vi "driveMotionProfile.vi"() -> ()   [LabVIEW 2018]
doc: "This VI is called for each TeleOp packet received from the DS where the robot is not disabled. It is often used to read from the joysticks and update I/O or to update setpoints for timed control loops. It should complete and return within 20 milliseconds or it may miss DS packets."
uses:
  Motion Profile SM.ctl
  <vilib>/Rock Robotics/WPI/ThirdParty/Phoenix-LabVIEW/Pigeon IMU/CTRE_PigeonIMU_CalibrationMode.ctl
  <vilib>/Rock Robotics/WPI/ThirdParty/Phoenix-LabVIEW/Motor Controller/Controls/CTRE_Phoenix_MotorControl_ControlMode.ctl
  <vilib>/Rock Robotics/WPI/ThirdParty/Phoenix-LabVIEW/Motor Controller/Controls/CTRE_Phoenix_MotorControl_MotionProfileControlMode.ctl
  <vilib>/Rock Robotics/WPI/Utilities/WPI_GetSetVariantRefNum.vi
  <vilib>/Rock Robotics/WPI/Joystick/WPI_JoystickArcadeMapping.vi
  <vilib>/Rock Robotics/WPI/ThirdParty/Phoenix-LabVIEW/Pigeon IMU/CTRE_PigeonIMU_GetFusedHeading.vi
  <vilib>/Rock Robotics/WPI/ThirdParty/Phoenix-LabVIEW/Pigeon IMU/CTRE_PigeonIMU_GetYPR.vi
  Constants.vi
  MotionProfileController.vi
panel:
  out "Fused Heading":T1
  out "Yaw Pitch Roll":cluster{"Yaw":dbl, "Pitch":dbl, "Roll":dbl}
  out "Waveform Chart":dbl(graph)
  out "MP File Ready":bool
  in  "Send Data Wait Time (ms)":u32
  in  "CSV File Name":string="Test_8ft"
  in  "Read File Wait Time (ms)":u32
  out "Save Tick Count":u32
  in  "Speed Limiter":dbl(slide)=1.0 scale=0.0..1.0
  out "Motion Profile SM":T2
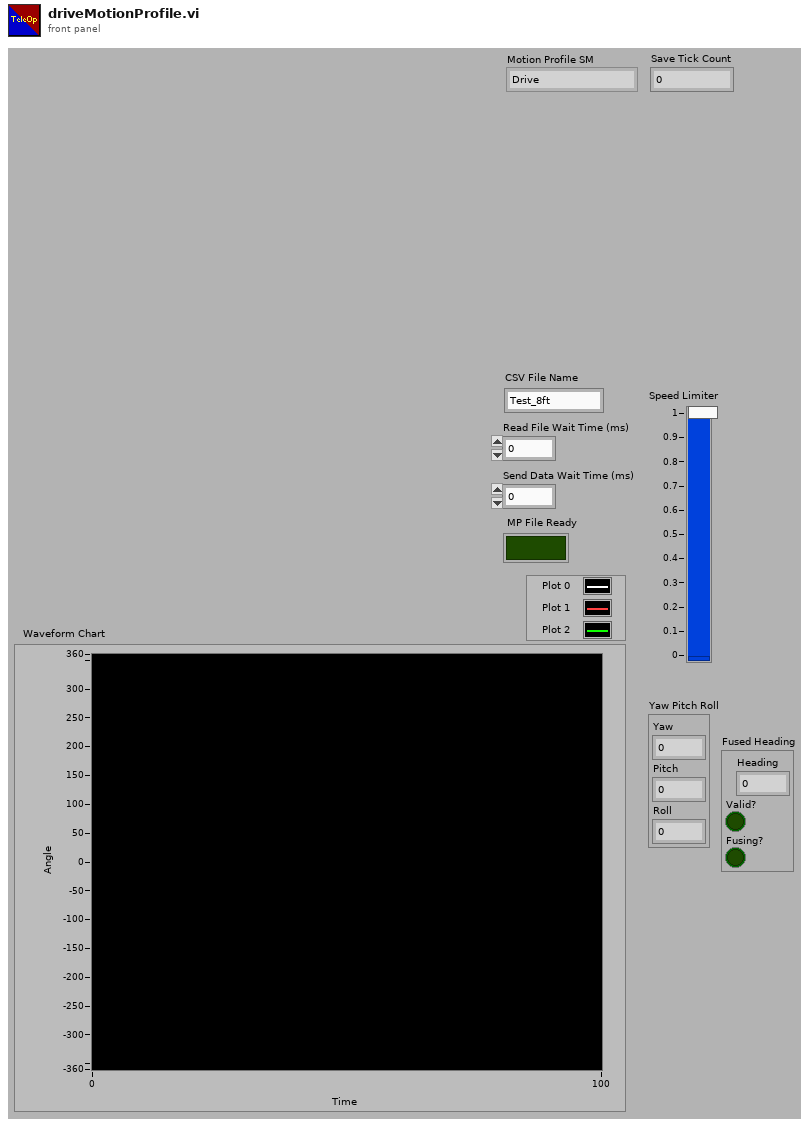
[diagram p1: front panel]
types:
  T1 = cluster{"Heading":dbl, "Valid?":bool, "Fusing?":bool}
  T2 = typedef "Motion Profile SM.ctl" = enum16{"Drive", "Reset Encoder", "Read File", "Send Data", "Motion Profile", "Wait for Release", "Set to Manual"}
  T3 = typedef "WPI_MotorControlDeviceRef.ctl" = cluster{"DeviceStatus":errorcluster, "Type":T4, "PWM":cluster{"PWM Channel":T5, "DeadBand":T6}, "CAN":cluster{"Device Number":u8, "SetOutput VI Ref":variant, "GetOutput VI Ref":variant, "Enable VI Ref":variant, "Disable VI Ref":variant, "Data":variant}, "Invert":bool, "DIO PWM":cluster{"PWM \"Enable\" Channel":T5, "DIOChannel":T7, "PWM Rate":dbl}}
  T4 = typedef "WPI_MotorControlType.ctl" = enum16{"PWM", "CAN", "DIO PWM"}
  T5 = typedef "FPGA_DIOPWMChannel.ctl" = enum8{"PWM 0", "PWM 1", "PWM 2", "PWM 3", "PWM 4", "PWM 5", "PWM 6", "PWM 7", "PWM 8", "PWM 9", "PWM MXP 0", "PWM MXP 1", "PWM MXP 2", "PWM MXP 3", "PWM MXP 4", "PWM MXP 5", "PWM MXP 6", "PWM MXP 7", "PWM MXP 8", "PWM MXP 9", "Invalid"}
  T6 = typedef "WPI_PWMDeadband.ctl" = cluster{"Name":string, "maxPositivePwm":i32, "minPositivePwm":i32, "centerPwm":i32, "maxNegativePwm":i32, "minNegativePwm":i32, "angularRange":u16}
  T7 = typedef "FPGA_DIOChannel.ctl" = enum8{"DIO 0", "DIO 1", "DIO 2", "DIO 3", "DIO 4", "DIO 5", "DIO 6", "DIO 7", "DIO 8", "DIO 9", "DIO MXP 0", "DIO MXP 1", "DIO MXP 2", "DIO MXP 3", "DIO MXP 4", "DIO MXP 5", "DIO MXP 6", "DIO MXP 7", "DIO MXP 8", "DIO MXP 9", "DIO MXP 10", "DIO MXP 11", "DIO MXP 12", "DIO MXP 13", "DIO MXP 14", "DIO MXP 15", "SPI Port CS1", "SPI Port CS2", "SPI Port CS3", "SPI Port MISO", "SPI Port MOSI", "Invalid"}
  T8 = typedef "WPI_JoystickDevRef.ctl" = cluster{"Device":T9}
  T9 = typedef "WPI_JoystickDeviceEnum.ctl" = enum16{"USB 0", "USB 1", "USB 2", "USB 3", "USB 4", "USB 5"}
  T10 = typedef "CTRE_PigeonIMU_DeviceRef.ctl" = cluster{"DeviceStatus":errorcluster, "Device Number":u8, "Type":T11, "Device ID":u32, "Handle":u64, "UsageFrame":u32, "Library Path":path}
  T11 = typedef "CTRE_PigeonIMU_ConnectionType.ctl" = u32
  T12 = typedef "CTRE_PigeonIMU_CalibrationMode.ctl" = u16
  T13 = cluster{"kP":dbl, "kI ":dbl, "kD":dbl, "kF":dbl, "I Zone":dbl, "Peak Out":dbl}
  T14 = enum16{"FollowerType_PercentOutput", "FollowerType_AuxOutput1"}
  T15 = typedef "CTRE_Phoenix_MotorControl_ControlMode.ctl" = u16
  T16 = typedef "CTRE_Phoenix_MotorControl_MotionProfileControlMode.ctl" = u16
  T17 = typedef "CTRE_Phoenix_MotorControl_BufferedTrajectoryPointStream_DeviceRef.ctl" = cluster{"Handle":u64, "Library Path":path}
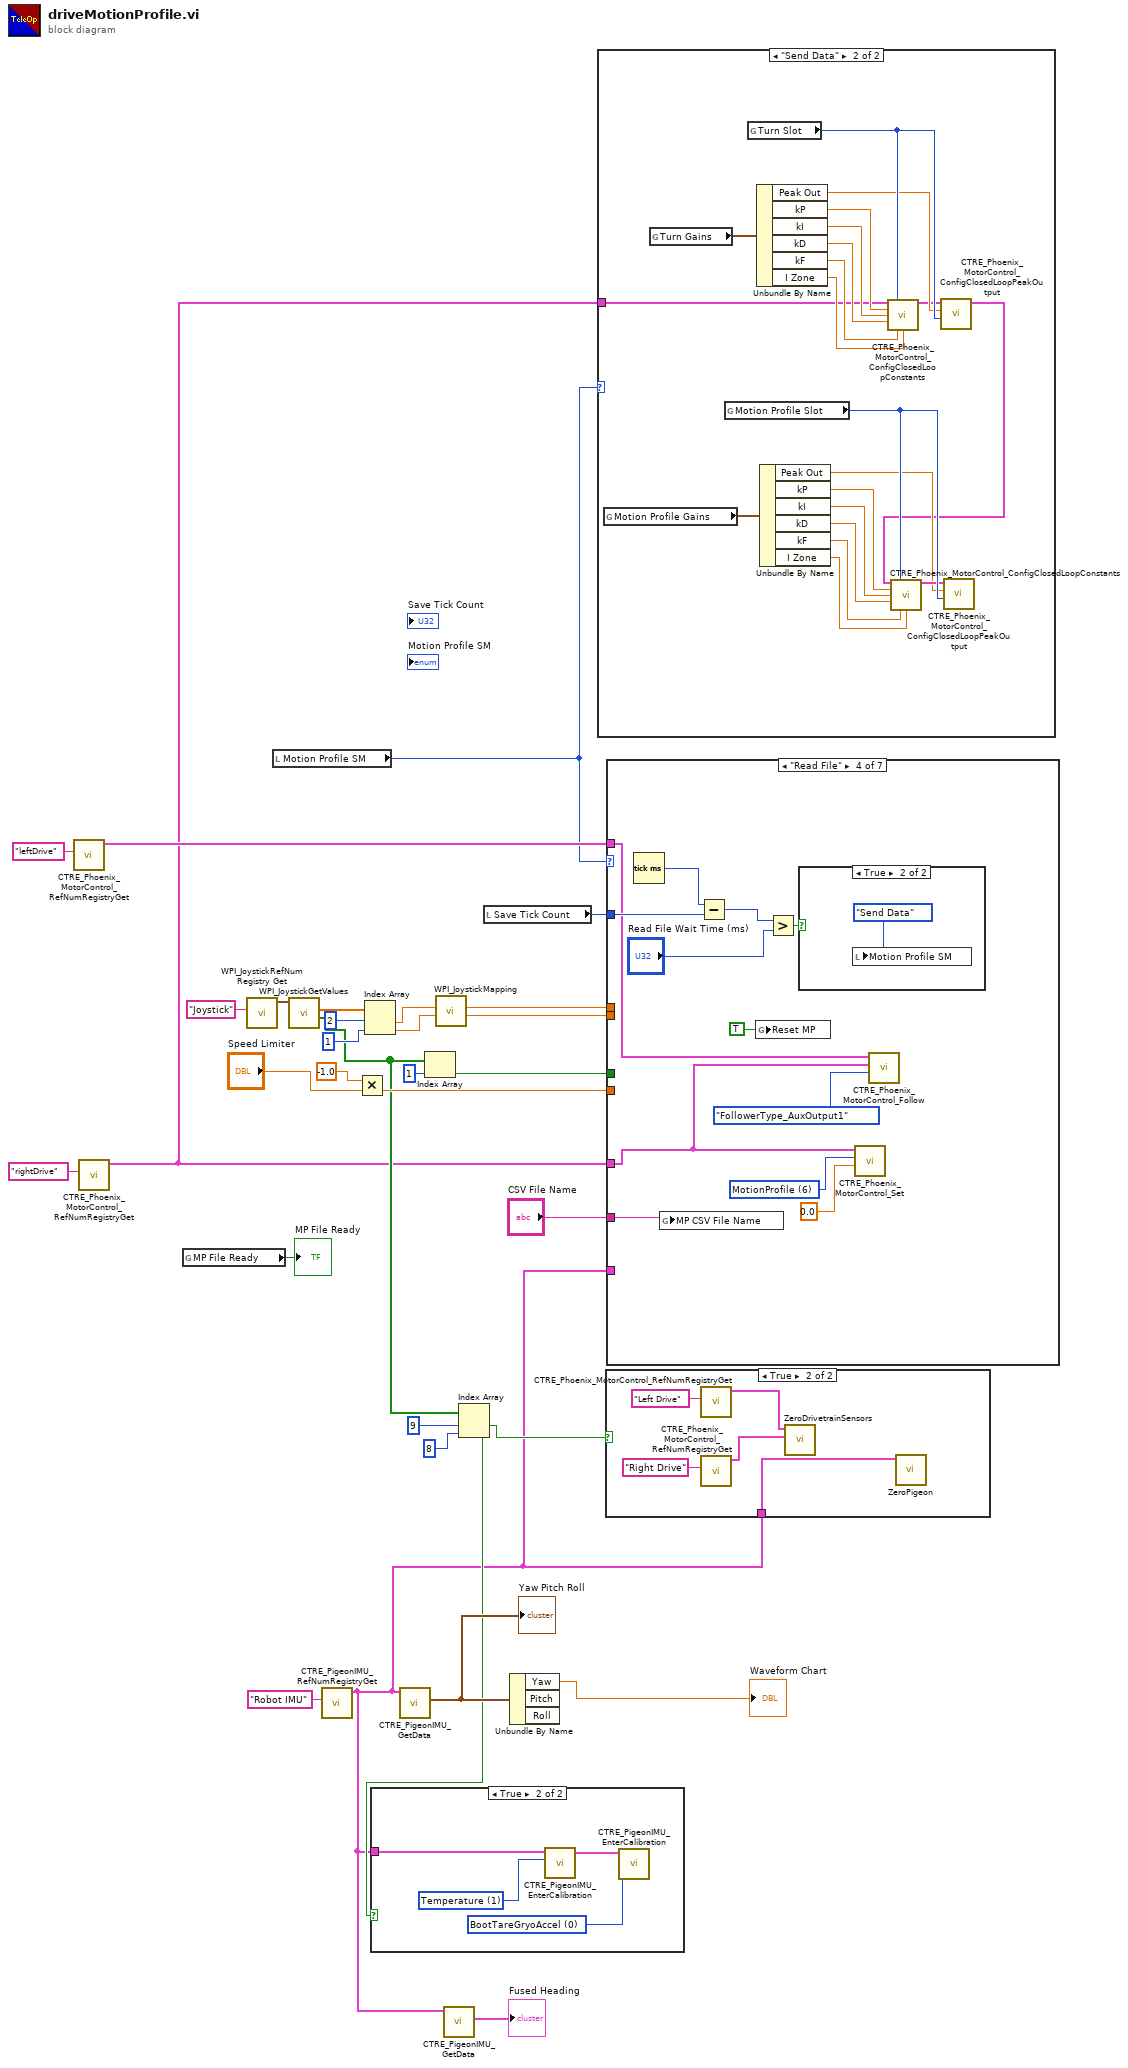
[diagram p0: block diagram]
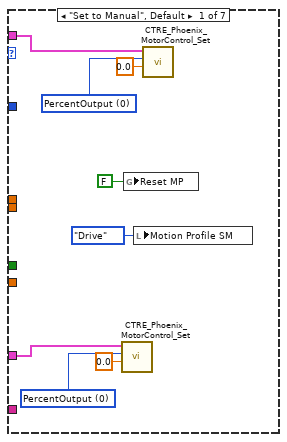
[diagram p5: hidden frame]
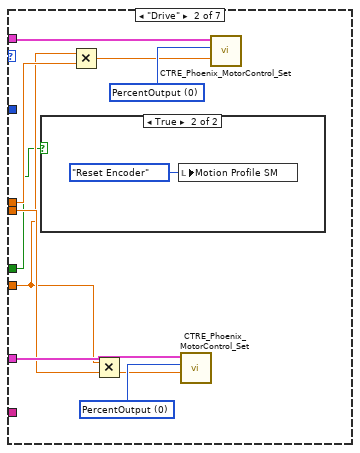
[diagram p6: hidden frame]
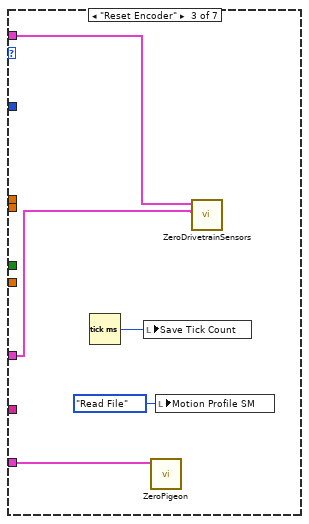
[diagram p8: hidden frame]
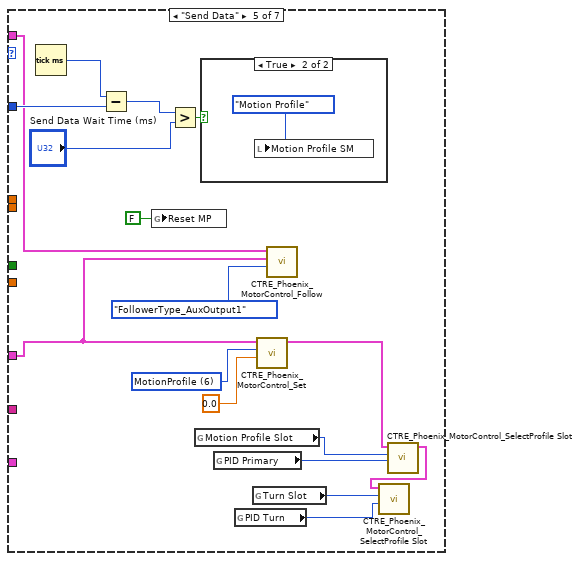
[diagram p10: hidden frame]
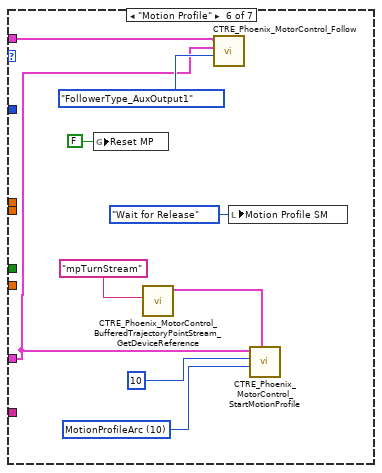
[diagram p12: hidden frame]
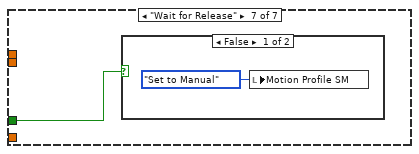
[diagram p13: hidden frame]
diagram:
  n1 = call <vilib>:"CTRE_Phoenix_MotorControl_RefNumRegistryGet.vi"("refnum name"="leftDrive") -> ("PhoenixMotorControlDevRef"=w14:T3)  [unwired: 9 in, 1 out]
  n2 = call <vilib>:"CTRE_Phoenix_MotorControl_RefNumRegistryGet.vi"("refnum name"="rightDrive") -> ("PhoenixMotorControlDevRef"=w4:T3)  [unwired: 9 in, 1 out]
  n3 = global read "MotionProfileController.vi" "MP File Ready"() -> (→"MP File Ready":bool)
  n4 = call <vilib>:"WPI_JoystickRefNum Registry Get.vi"("refnum name"="Joystick") -> ("JoystickDevRef"=w30:T8)  [unwired: 1 in, 9 out]
  n5 = local read "Motion Profile SM"() -> (w3:T2)
  n6 = call <vilib>:"WPI_JoystickGetValues.vi"("JoystickDevRef"=w30) -> ("Buttons"=w12:bool[], "Axes"=w27:dbl[])  [unwired: 6 in, 3 out]
  n7 = call <vilib>:"CTRE_PigeonIMU_RefNumRegistryGet.vi"("refnum name"="Robot IMU") -> ("PigeonIMUDevRef"=w2:T10)  [unwired: 9 in, 1 out]
  n8 = Multiply(x=-1.0, y="Speed Limiter") -> (x*y=w24:dbl)
  n9 = Index Array(array=w27, index #1=2 ("index"), index #2=1 ("index")) -> (element #1=w20:dbl, element #2=w19:dbl)
  n10 = call-poly <vilib>:"CTRE_PigeonIMU_GetData.vi"("PigeonIMUDevRef"=w2) -> ("Yaw Pitch Roll"=w8:cluster{"Yaw":dbl, "Pitch":dbl, "Roll":dbl})  [unwired: 8 in, 2 out]
  "Yaw Pitch Roll" <- w8
  n11 = Index Array(array=w12, index=1) -> (element=w21:bool)
  n12 = call-poly <vilib>:"WPI_JoystickMapping.vi"("Y axis value"=w19, "X axis value"=w20) -> ("Right Motor Value"=w17:dbl, "Left Motor Value"=w18:dbl)  [unwired: 8 in]
  n13 = call-poly <vilib>:"CTRE_PigeonIMU_GetData.vi"("PigeonIMUDevRef"=w2) -> ("Fused Heading"=→"Fused Heading":T1)  [unwired: 8 in, 2 out]
  n14 = Index Array(array=w12, index #1=9 ("index"), index #2=8 ("index")) -> (element #1=w13:bool, element #2=w6:bool)
  n15 = case shown="True" w6 {
    tunnel: w2 -> [_ w36]
    frame False {
    }
    frame True {
      w33 = T12 0 items=["BootTareGryoAccel"=0, "Temperature"=1, "Magnetometer12Pt"=2, "Magnetometer360"=3, "Accelerometer"=5] ("CalibrationMode")
      w35 = T12 1 items=["BootTareGryoAccel"=0, "Temperature"=1, "Magnetometer12Pt"=2, "Magnetometer360"=3, "Accelerometer"=5] ("CalibrationMode")
      n16 = call <vilib>:"CTRE_PigeonIMU_EnterCalibration.vi"("CalibrationMode"=w35, "PigeonIMUDevRef"=w36) -> ("PigeonIMUDevRef"=w34:T10)  [unwired: 8 in, 1 out]
      n17 = call <vilib>:"CTRE_PigeonIMU_EnterCalibration.vi"("CalibrationMode"=w33, "PigeonIMUDevRef"=w34) -> ()  [unwired: 8 in, 2 out]
    }
  }
  n18 = local read "Save Tick Count"() -> (w16:u32)
  n19 = Unbundle By Name(w8) -> ("Yaw"=→"Waveform Chart":dbl)  [unwired: 2 out]
  n20 = case shown="\"Send Data\"" w3 {
    tunnel: w4 -> [_ w37]
    frame "Drive", Default {
    }
    frame "Send Data" {
      n21 = global read "Constants.vi" "Motion Profile Gains"() -> (w46:T13)
      n22 = global read "Constants.vi" "Turn Gains"() -> (w47:T13)
      n23 = global read "Constants.vi" "Motion Profile Slot"() -> (w55:i32)
      n24 = global read "Constants.vi" "Turn Slot"() -> (w56:i32)
      n25 = Unbundle By Name(w47) -> ("Peak Out"=w54:dbl, "kP"=w48:dbl, "kI"=w49:dbl, "kD"=w50:dbl, "kF"=w51:dbl, "I Zone"=w52:dbl)
      n26 = Unbundle By Name(w46) -> ("Peak Out"=w39:dbl, "kP"=w45:dbl, "kI"=w44:dbl, "kD"=w43:dbl, "kF"=w42:dbl, "I Zone"=w41:dbl)
      n27 = call <vilib>:"CTRE_Phoenix_MotorControl_ConfigClosedLoopConstants.vi"("PhoenixMotorControlDevRef"=w37, "slotIdx"=w56, "P"=w48, "I"=w49, "D"=w50, "F"=w51, "I Zone"=w52) -> ("PhoenixMotorControlDevRef"=w53:T3)  [unwired: 7 in, 1 out]
      n28 = call <vilib>:"CTRE_Phoenix_MotorControl_ConfigClosedLoopPeakOutput.vi"("slotIdx"=w56, "peakOutput"=w54, "PhoenixMotorControlDevRef"=w53) -> ("PhoenixMotorControlDevRef"=w38:T3)  [unwired: 7 in, 1 out]
      n29 = call <vilib>:"CTRE_Phoenix_MotorControl_ConfigClosedLoopConstants.vi"("PhoenixMotorControlDevRef"=w38, "slotIdx"=w55, "P"=w45, "I"=w44, "D"=w43, "F"=w42, "I Zone"=w41) -> ("PhoenixMotorControlDevRef"=w40:T3)  [unwired: 7 in, 1 out]
      n30 = call <vilib>:"CTRE_Phoenix_MotorControl_ConfigClosedLoopPeakOutput.vi"("slotIdx"=w55, "peakOutput"=w39, "PhoenixMotorControlDevRef"=w40) -> ()  [unwired: 7 in, 2 out]
    }
  }
  n31 = case shown="True" w13 {
    tunnel: w2 -> [_ w57]
    frame False {
    }
    frame True {
      n32 = call <vilib>:"CTRE_Phoenix_MotorControl_RefNumRegistryGet.vi"("refnum name"="Left Drive") -> ("PhoenixMotorControlDevRef"=w58:T3)  [unwired: 9 in, 1 out]
      n33 = call <vilib>:"CTRE_Phoenix_MotorControl_RefNumRegistryGet.vi"("refnum name"="Right Drive") -> ("PhoenixMotorControlDevRef"=w59:T3)  [unwired: 9 in, 1 out]
      n34 = call "ZeroDrivetrainSensors.vi"("Talon 2"=w59, "Talon 1"=w58) -> ()  [unwired: 8 in, 2 out]
      n35 = call "ZeroPigeon.vi"("Pigeon"=w57) -> ()  [unwired: 8 in, 1 out]
    }
  }
  n36 = case shown="\"Read File\"" w3 {
    tunnel: w14 -> [w68 w78 w82 w87 w106 w124 _]
    tunnel: w4 -> [w66 w76 w83 w86 w105 w122 _]
    tunnel: w18 -> [_ w75 _ _ _ _ _]
    tunnel: w17 -> [_ w74 _ _ _ _ _]
    tunnel: w24 -> [_ w71 _ _ _ _ _]
    tunnel: w21 -> [_ w70 _ _ _ _ w126]
    tunnel: w16 -> [_ _ _ w96 w114 _ _]
    tunnel: "CSV File Name" -> [_ _ _ w89 _ _ _]
    tunnel: w2 -> [_ _ w81 _ _ _ _]
    frame "Set to Manual", Default {
      w67 = T15 0 items=["PercentOutput"=0, "Position"=1, "Velocity"=2, "Current"=3, "Follower"=5, "MotionProfile"=6, "MotionMagic"=7, "MotionMagicArc"=8, "MotionProfileArc"=10, "Disabled"=15] ("Control Mode")
      w69 = T15 0 items=["PercentOutput"=0, "Position"=1, "Velocity"=2, "Current"=3, "Follower"=5, "MotionProfile"=6, "MotionMagic"=7, "MotionMagicArc"=8, "MotionProfileArc"=10, "Disabled"=15] ("Control Mode")
      n37 = call <vilib>:"CTRE_Phoenix_MotorControl_Set.vi"("Output"=0.0, "Control Mode"=w67, "PhoenixMotorControlDevRef"=w66) -> ()  [unwired: 7 in, 2 out]
      n38 = global write "MotionProfileController.vi" "Reset MP"(FALSE ("Reset Motion Profile Points")) -> ()
      n39 = local write "Motion Profile SM"(Motion_Profile_SM."Drive" ("Motion Profile SM")) -> ()
      n40 = call <vilib>:"CTRE_Phoenix_MotorControl_Set.vi"("Output"=0.0, "Control Mode"=w69, "PhoenixMotorControlDevRef"=w68) -> ()  [unwired: 7 in, 2 out]
    }
    frame "Drive" {
      w77 = T15 0 items=["PercentOutput"=0, "Position"=1, "Velocity"=2, "Current"=3, "Follower"=5, "MotionProfile"=6, "MotionMagic"=7, "MotionMagicArc"=8, "MotionProfileArc"=10, "Disabled"=15] ("Control Mode")
      w79 = T15 0 items=["PercentOutput"=0, "Position"=1, "Velocity"=2, "Current"=3, "Follower"=5, "MotionProfile"=6, "MotionMagic"=7, "MotionMagicArc"=8, "MotionProfileArc"=10, "Disabled"=15] ("Control Mode")
      n41 = case shown="True" w70 {
        frame False {
        }
        frame True {
          n42 = local write "Motion Profile SM"(Motion_Profile_SM."Reset Encoder" ("Motion Profile SM")) -> ()
        }
      }
      n43 = Multiply(x=w71, y=w75) -> (x*y=w73:dbl)
      n44 = Multiply(x=w71, y=w74) -> (x*y=w72:dbl)
      n45 = call <vilib>:"CTRE_Phoenix_MotorControl_Set.vi"("Output"=w72, "Control Mode"=w77, "PhoenixMotorControlDevRef"=w76) -> ()  [unwired: 7 in, 2 out]
      n46 = call <vilib>:"CTRE_Phoenix_MotorControl_Set.vi"("Output"=w73, "Control Mode"=w79, "PhoenixMotorControlDevRef"=w78) -> ()  [unwired: 7 in, 2 out]
    }
    frame "Reset Encoder" {
      n47 = Tick Count (ms)() -> (millisecond timer value=w84:u32)
      n48 = local write "Save Tick Count"(w84) -> ()
      n49 = call "ZeroPigeon.vi"("Pigeon"=w81) -> ()  [unwired: 8 in, 1 out]
      n50 = local write "Motion Profile SM"(Motion_Profile_SM."Read File" ("Motion Profile SM")) -> ()
      n51 = call "ZeroDrivetrainSensors.vi"("Talon 2"=w83, "Talon 1"=w82) -> ()  [unwired: 8 in, 2 out]
    }
    frame "Read File" {
      w92 = T15 6 items=["PercentOutput"=0, "Position"=1, "Velocity"=2, "Current"=3, "Follower"=5, "MotionProfile"=6, "MotionMagic"=7, "MotionMagicArc"=8, "MotionProfileArc"=10, "Disabled"=15] ("Control Mode")
      n52 = Tick Count (ms)() -> (millisecond timer value=w97:u32)
      n53 = global write "MotionProfileController.vi" "MP CSV File Name"(w89) -> ()
      n54 = Subtract(x=w97, y=w96) -> (x-y=w95:u32)
      n55 = global write "MotionProfileController.vi" "Reset MP"(TRUE ("Reset Motion Profile Points")) -> ()
      n56 = Greater?(x=w95, y="Read File Wait Time (ms)") -> (0:w93:bool)
      n57 = case shown="True" w93 {
        frame False {
        }
        frame True {
          n58 = local write "Motion Profile SM"(Motion_Profile_SM."Send Data" ("Motion Profile SM")) -> ()
        }
      }
      n59 = call <vilib>:"CTRE_Phoenix_MotorControl_Set.vi"("Output"=0.0, "Control Mode"=w92, "PhoenixMotorControlDevRef"=w86) -> ()  [unwired: 7 in, 2 out]
      n60 = call <vilib>:"CTRE_Phoenix_MotorControl_Follow.vi"("FollowerType"=T14."FollowerType_AuxOutput1", "Master Controller to Follow"=w86, "PhoenixMotorControlDevRef"=w87) -> ()  [unwired: 7 in, 2 out]
    }
    frame "Send Data" {
      w110 = T15 6 items=["PercentOutput"=0, "Position"=1, "Velocity"=2, "Current"=3, "Follower"=5, "MotionProfile"=6, "MotionMagic"=7, "MotionMagicArc"=8, "MotionProfileArc"=10, "Disabled"=15] ("Control Mode")
      n61 = Tick Count (ms)() -> (millisecond timer value=w115:u32)
      n62 = Subtract(x=w115, y=w114) -> (x-y=w113:u32)
      n63 = global write "MotionProfileController.vi" "Reset MP"(FALSE ("Reset Motion Profile Points")) -> ()
      n64 = Greater?(x=w113, y="Send Data Wait Time (ms)") -> (0:w111:bool)
      n65 = global read "Constants.vi" "Motion Profile Slot"() -> (w103:i32)
      n66 = case shown="True" w111 {
        frame False {
        }
        frame True {
          n67 = local write "Motion Profile SM"(Motion_Profile_SM."Motion Profile" ("Motion Profile SM")) -> ()
        }
      }
      n68 = global read "Constants.vi" "PID Primary"() -> (w104:i32)
      n69 = global read "Constants.vi" "PID Turn"() -> (w100:i32)
      n70 = global read "Constants.vi" "Turn Slot"() -> (w101:i32)
      n71 = call <vilib>:"CTRE_Phoenix_MotorControl_Set.vi"("Output"=0.0, "Control Mode"=w110, "PhoenixMotorControlDevRef"=w105) -> ("PhoenixMotorControlDevRef"=w99:T3)  [unwired: 7 in, 1 out]
      n72 = call <vilib>:"CTRE_Phoenix_MotorControl_Follow.vi"("FollowerType"=T14."FollowerType_AuxOutput1", "Master Controller to Follow"=w105, "PhoenixMotorControlDevRef"=w106) -> ()  [unwired: 7 in, 2 out]
      n73 = call <vilib>:"CTRE_Phoenix_MotorControl_SelectProfile Slot.vi"("pidLoopIdx"=w104, "slotIdx"=w103, "PhoenixMotorControlDevRef"=w99) -> ("PhoenixMotorControlDevRef"=w102:T3)  [unwired: 7 in, 1 out]
      n74 = call <vilib>:"CTRE_Phoenix_MotorControl_SelectProfile Slot.vi"("pidLoopIdx"=w100, "slotIdx"=w101, "PhoenixMotorControlDevRef"=w102) -> ()  [unwired: 7 in, 2 out]
    }
    frame "Motion Profile" {
      w121 = T16 10 items=["MotionProfile"=6, "MotionProfileArc"=10] ("Control Mode")
      n75 = global write "MotionProfileController.vi" "Reset MP"(FALSE ("Reset Motion Profile Points")) -> ()
      n76 = call <vilib>:"CTRE_Phoenix_MotorControl_BufferedTrajectoryPointStream_GetDeviceReference.vi"("refnum name"="mpTurnStream") -> ("BufferedTrajectoryPointStream_DevRef"=w118:T17)  [unwired: 9 in, 1 out]
      n77 = call <vilib>:"CTRE_Phoenix_MotorControl_Follow.vi"("FollowerType"=T14."FollowerType_AuxOutput1", "Master Controller to Follow"=w122, "PhoenixMotorControlDevRef"=w124) -> ()  [unwired: 7 in, 2 out]
      n78 = local write "Motion Profile SM"(Motion_Profile_SM."Wait for Release" ("Motion Profile SM")) -> ()
      n79 = call <vilib>:"CTRE_Phoenix_MotorControl_StartMotionProfile.vi"("BufferedTrajectoryPointStream_DevRef"=w118, "Control Mode"=w121, "minBufferedPts"=u32 10, "PhoenixMotorControlDevRef"=w122) -> ()  [unwired: 6 in, 2 out]
    }
    frame "Wait for Release" {
      n80 = case shown="False" w126 {
        frame False {
          n81 = local write "Motion Profile SM"(Motion_Profile_SM."Set to Manual" ("Motion Profile SM")) -> ()
        }
        frame True {
        }
      }
    }
  }
